vi "sio AbortRead.vi"(11 "port":i32) -> (0 "Status":i32, 3 "port":i32)   [LabVIEW 2015, in "PCOMM.lvlib"]
doc: "int WINAPI sio_AbortRead(int port);\n中断读操作"
uses:
  PCOMM.lvlib
  PCOMM.DLL
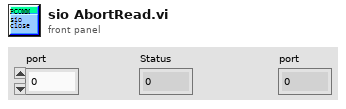
[diagram p1: front panel]
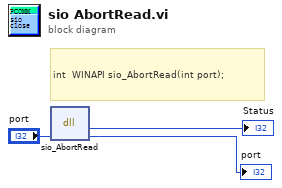
[diagram p0: block diagram]
diagram:
  # "int  WINAPI sio_AbortRead(int port);"
  n1 = dll-call lib="PTH2^abs EDesktopLabview串口助手串口助手2.0Ing10_v3.2.0SubVIpcomm库PCOMM.*" fn="sio_AbortRead"("port"="port") -> ("Status"=→"Status":i32, "port"=→"port":i32)  [unwired: 3 in, 2 out]
